vi "setHeater.vi"(6 "Channel":i32, 8 "error in (no error)":errorcluster, 10 "Current (A)":dbl, 11 "Instrument.Cryostat in":refnum<class "Instrument.Cryostat.lvclass">) -> (0 "error out":errorcluster, 3 "Instrument.Cryostat out":refnum<class "Instrument.Cryostat.lvclass">)   [LabVIEW 2019, in "Instrument.Cryostat.lvclass"]
uses:
  Instrument.Cryostat.lvclass
  C:/Users/patrick/Documents/GitHub/Instrument-Framework/lvsrc/Instrument/Instrument.lvclass
  Typedefs/setHeater--cluster.ctl
  Instrument/Instrument.lvclass/Instrument.ctl
  6e4c65a3-0cfa-4c3a-bc5f-3524f17930a2.vi
  6e4c65a3-0cfa-4c3a-bc5f-3524f17930a2.vi/627e8be8-a4ac-433c-aabd-789326c97fd9.vi
  6e4c65a3-0cfa-4c3a-bc5f-3524f17930a2.vi/4649e7dd-cce8-4ac4-b322-0a98d84f2fcb.vi
  Instrument/Private/Get Client Type.vi
  6e4c65a3-0cfa-4c3a-bc5f-3524f17930a2.vi/627e8be8-a4ac-433c-aabd-789326c97fd9.vi/d73feb51-6d65-494b-8cbe-05dd9a956011.vi
  6e4c65a3-0cfa-4c3a-bc5f-3524f17930a2.vi/627e8be8-a4ac-433c-aabd-789326c97fd9.vi/80eff681-d9d8-4cba-97be-633cf55270bc.vi
  Instrument/Private/Set Dependencies.vi
  6e4c65a3-0cfa-4c3a-bc5f-3524f17930a2.vi/4649e7dd-cce8-4ac4-b322-0a98d84f2fcb.vi/aee261c7-bc68-4494-92a1-ae27f0a00f87.vi
  6e4c65a3-0cfa-4c3a-bc5f-3524f17930a2.vi/4649e7dd-cce8-4ac4-b322-0a98d84f2fcb.vi/42e175e4-a5b8-495a-a3ec-68a150131f74.vi
  6e4c65a3-0cfa-4c3a-bc5f-3524f17930a2.vi/4649e7dd-cce8-4ac4-b322-0a98d84f2fcb.vi/d8b8bc0a-df33-44be-8b12-256a022b0822.vi
  6e4c65a3-0cfa-4c3a-bc5f-3524f17930a2.vi/627e8be8-a4ac-433c-aabd-789326c97fd9.vi/80eff681-d9d8-4cba-97be-633cf55270bc.vi/0b2e8f7d-cfc9-4fe5-a21e-0777c31258e6.vi
  6e4c65a3-0cfa-4c3a-bc5f-3524f17930a2.vi/627e8be8-a4ac-433c-aabd-789326c97fd9.vi/80eff681-d9d8-4cba-97be-633cf55270bc.vi/30df1777-6ab1-49b8-a34a-3c1650ee933f.vi
  6e4c65a3-0cfa-4c3a-bc5f-3524f17930a2.vi/4649e7dd-cce8-4ac4-b322-0a98d84f2fcb.vi/42e175e4-a5b8-495a-a3ec-68a150131f74.vi/9ee4ccb0-b27b-403d-8253-52a56cd6028b.vi
  6e4c65a3-0cfa-4c3a-bc5f-3524f17930a2.vi/4649e7dd-cce8-4ac4-b322-0a98d84f2fcb.vi/42e175e4-a5b8-495a-a3ec-68a150131f74.vi/cfd53a0e-a313-4ab7-8bcc-18b76d2cae70.vi
  6e4c65a3-0cfa-4c3a-bc5f-3524f17930a2.vi/4649e7dd-cce8-4ac4-b322-0a98d84f2fcb.vi/d8b8bc0a-df33-44be-8b12-256a022b0822.vi/dc073bcd-5ace-412f-8e4a-4838771d015f.vi
  6e4c65a3-0cfa-4c3a-bc5f-3524f17930a2.vi/4649e7dd-cce8-4ac4-b322-0a98d84f2fcb.vi/d8b8bc0a-df33-44be-8b12-256a022b0822.vi/ad5222c0-3d0c-4c8c-b228-051d507c9696.vi
  Instrument/Private/Get RC Connection Status.vi
  Instrument/Private/Get Dependencies.vi
  <userlib>/LevyLab/RemoteControl/API/Send and Receive.vi
  <vilib>/Utility/Data Type/Get Type Information.vi
  <vilib>/JDP Science/JSONtext/JSON text to Variant.vi
  Instrument/API/Instrument.GetPublicEvents.vi
  <vilib>/JDP Science/JSONtext/Variant to JSON Text.vi
  <vilib>/National Instruments/GUID Generator/Guid Generator.vi
  Instrument/API/Instrument.sendMessageToProcess.vi
  Instrument/Private/Instrument.MessageFromProcess.EventStructure.vi
  <vilib>/JDP Science/JSONtext/LVClass Serializer/JSONtext LVClass Serializer.lvclass
  Instrument/Instrument.lvclass
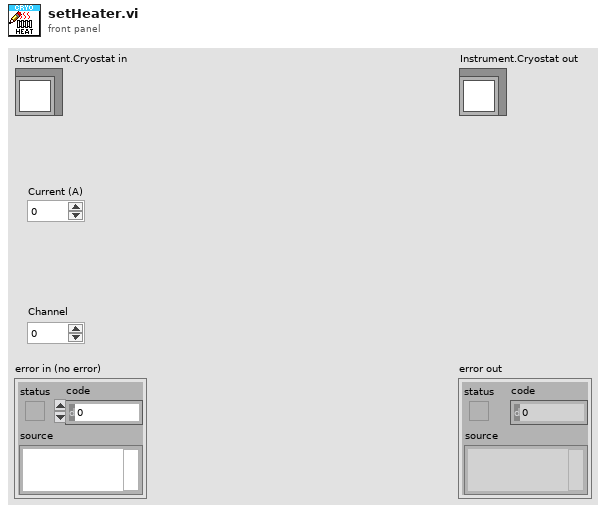
[diagram p1: front panel]
types:
  T1 = typedef "Instrument.Cryostat.lvclass/setHeater--cluster.ctl" = cluster{"Channel":i32, "Current":dbl}
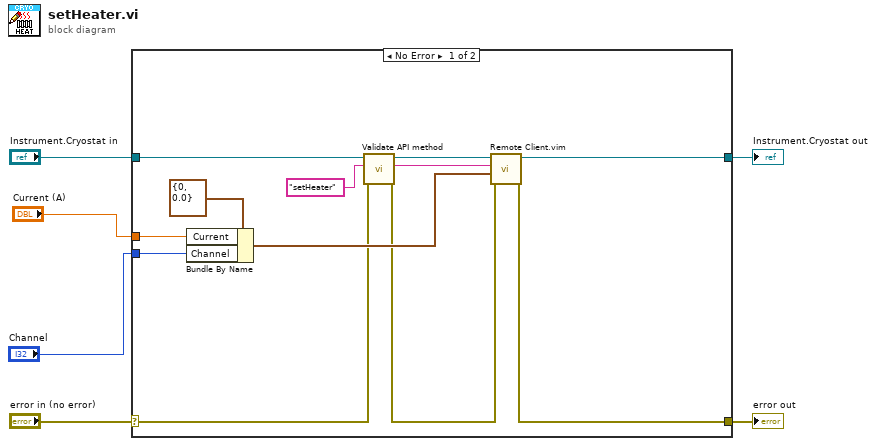
[diagram p0: block diagram]
diagram:
  n1 = case shown="No Error" "error in (no error)" {
    selector: "error in (no error)" -> [w8 w20]
    tunnel: [w7 w20] -> w5
    tunnel: [w10 w19] -> w3
    tunnel: "Instrument.Cryostat in" -> [w12 w19]
    tunnel: "Current (A)" -> [w18 _]
    tunnel: "Channel" -> [w17 _]
    frame No Error {
      n2 = Bundle By Name(cluster=T1 {"Channel"=0, "Current"=0.0} ("Set Temperature"), "Current"=w18, "Channel"=w17) -> (w11:T1)
      n3 = call "Validate API method.vi"("error in (no error)"=w8, "command in"="setHeater" ("error message (\"\")"), "Instrument in"=w12) -> ("error out"=w9:errorcluster, "command out"=w14:string, "Instrument out"=w13:refnum<class "Instrument.Cryostat.lvclass">)  [unwired: 6 in]
      n4 = call "Remote Client.vim"("error in (no error)"=w9, "params"=w11, "method"=w14, "Instrument in"=w13) -> ("error out"=w7:errorcluster, "Instrument out"=w10:refnum<class "Instrument.Cryostat.lvclass">)  [unwired: 4 in, 2 out]
    }
    frame Error {
    }
  }
  "error out" <- w5
  "Instrument.Cryostat out" <- w3
